vi "Initialize.vi"(8 "error in (no error)":errorcluster, 11 "Camera in":refnum<class "Camera.lvclass">) -> (0 "error out":errorcluster, 3 "Camera out":refnum<class "Camera.lvclass">)   [LabVIEW 2020, in "Camera.lvlib" / "Camera.lvclass"]
uses:
  Camera.lvclass
  <vilib>/ActorFramework/Actor/Actor.lvclass
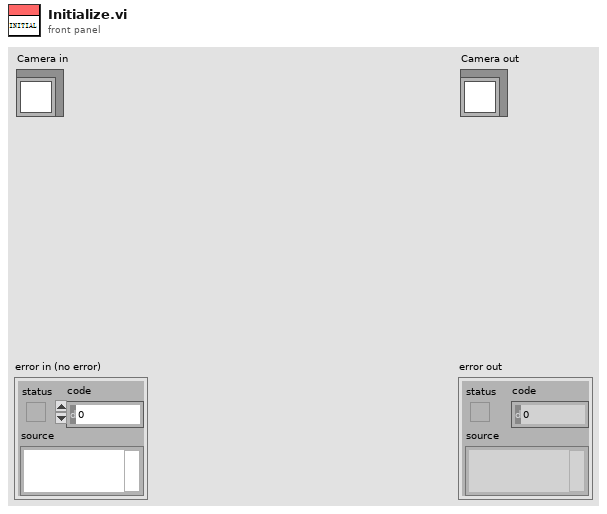
[diagram p1: front panel]
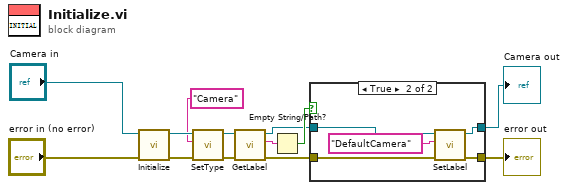
[diagram p0: block diagram]
diagram:
  n1 = call-parent "Initialize.vi"("error in (no error)"="error in (no error)", "Device in"="Camera in") -> ("error out"=w13:errorcluster, "Device out"=w9:refnum<class "Camera.lvclass">)  [unwired: 8 in]
  n2 = call-dynamic "SetType.vi"("error in (no error)"=w13, "Type"="Camera", "GRMActor in"=w9) -> ("error out"=w10:errorcluster, "GRMActor out"=w7:refnum<class "Camera.lvclass">)  [unwired: 7 in]
  n3 = call-dynamic "GetLabel.vi"("error in (no error)"=w10, "GRMActor in"=w7) -> ("error out"=w3:errorcluster, "Label"=w6:string, "GRMActor out"=w4:refnum<class "Camera.lvclass">)  [unwired: 7 in]
  n4 = Empty String/Path?(string/path=w6) -> (empty?=w5:bool)
  n5 = case shown="True" w5 {
    tunnel: w4 -> [w15 w18]
    tunnel: w3 -> [w14 w20]
    tunnel: [w15 w17] -> w2
    tunnel: [w14 w19] -> w1
    frame False {
    }
    frame True {
      n6 = call-dynamic "SetLabel.vi"("error in (no error)"=w20, "Label"="DefaultCamera", "GRMActor in"=w18) -> ("error out"=w19:errorcluster, "GRMActor out"=w17:refnum<class "Camera.lvclass">)  [unwired: 7 in]
    }
  }
  "error out" <- w1
  "Camera out" <- w2
